vi "Start.vi"(8 "error in (no error)":errorcluster, 10 "Container":refnum<vi>, 11 "ArrayManager in":refnum<class "ArrayManager.lvclass">) -> (0 "error out":errorcluster, 3 "ArrayManager out":refnum<class "ArrayManager.lvclass">)   [LabVIEW 2020, in "OOPanel.lvlib" / "ArrayManager.lvclass"]
uses:
  ArrayManager.lvclass
  ArrayManager.lvclass/ArrayManager.ctl
  Array Panel Async.vi
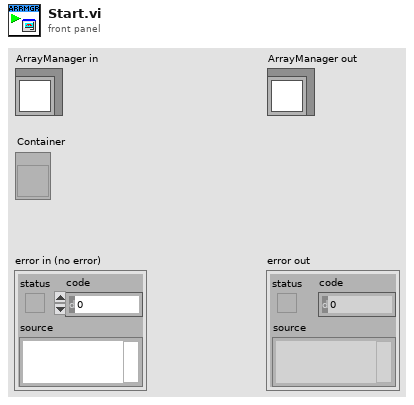
[diagram p1: front panel]
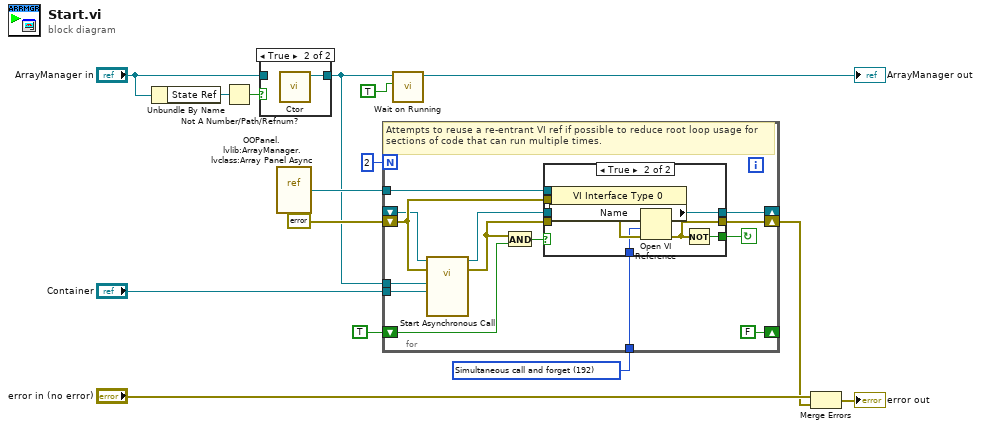
[diagram p0: block diagram]
diagram:
  w6 = 192 items=["Record modifications"=1, "Open templates for editing"=2, "Prompt user to save"=4, "Prepare for reentrant run"=8, "Prompt to find missing subVIs"=16, "Hide loading dialog box"=32, "Enable simultaneous calls"=64, "Prepare to call and forget"=128, "Simultaneous call and forget"=192, "Prepare to call and collect"=256, "Simultaneous call and collect"=320]
  n1 = Unbundle By Name("ArrayManager in") -> ("State Ref"=w11:refnum<data-value>)
  n2 = Not A Number/Path/Refnum?(number/path/refnum=w11) -> (NaN/Path/Refnum?=w10:bool)
  n3 = case shown="True" w10 {
    tunnel: "ArrayManager in" -> [w16 _]
    tunnel: [w16 w17] -> w4
    frame False {
    }
    frame True {
      n4 = call "Ctor.vi"() -> ("PanelArray"=w17:refnum<class "ArrayManager.lvclass">)  [unwired: 10 in, 1 out]
    }
  }
  n5 = vi-ref "OOPanel.lvlib:ArrayManager.lvclass:Array Panel Async.vi"() -> (w5:refnum<vi>)
  n6 = for {
    N: 2 -> [_]
    tunnel: w5 -> [w30]
    tunnel: w6 -> [w29]
    shift-right: [w28] -> _
    shift-left: _ -> [w27]
    shift-right: [w25] -> w2
    shift-left: errorcluster {"status"=FALSE, "code"=0, "source"=""} ("error constant") -> [w31]
    shift-right: [FALSE] -> _
    shift-left: TRUE -> [w22]
    tunnel: w4 -> [w19]
    tunnel: "Container" -> [w18]
    stop <- w21 continue-if-true
    # "Attempts to reuse a re-entrant VI ref if possible to reduce root loop usage for sections of code that can run multiple times."
    n7 = call-by-ref "Start Asynchronous Call"(reference=w27, error in=w31, "Container"=w18, "PanelArray in"=w19) -> (reference out=w26:refnum<vi>, error out=w24:errorcluster)  [unwired: 10 in]
    n8 = And(x=w24, y=w22) -> (x .and. y?=w23:bool)
    n9 = case shown="True" w23 {
      tunnel: w30 -> [_ w41]
      tunnel: w29 -> [_ w39]
      tunnel: [w33 w37] -> w28
      tunnel: w26 -> [w33 _]
      tunnel: [w32 w35] -> w25
      tunnel: w24 -> [w32 _]
      tunnel: w31 -> [_ w36]
      tunnel: [_ w34] -> w21
      frame False {
      }
      frame True {
        n10 = property class="VI Interface Type 0"(reference=w41, error in=w36) -> (reference out=w38:refnum<vi>, error out=w42:errorcluster, "Name"=w40:string)
        n11 = Open VI Reference(type specifier VI Refnum (for type only)=w38, vi path=w40, options=w39, error in (no error)=w42) -> (vi reference=w37:refnum<vi>, error out=w35:errorcluster)  [unwired: 2 in]
        n12 = Not(x=w35) -> (.not. x?=w34:bool)
      }
    }
  }
  n13 = call "Wait on Running.vi"("Value"=TRUE, "ArrayManager in"=w4) -> ("ArrayManager out"=→"ArrayManager out":refnum<class "ArrayManager.lvclass">)  [unwired: 8 in, 1 out]
  n14 = Merge Errors("error in (no error)", w2) -> (→"error out":errorcluster)
